vi "CPU_IRQ_handle.vi"(11 "registers":T1 {"P" format="%08b"; "PC" format="%04x"; "SP" format="%02x"; "Y" format="%02x"; "X" format="%02x"; "A" format="%02x"}) -> (3 "registers":T1 {"P" format="%08b"; "PC" format="%04x"; "SP" format="%02x"; "Y" format="%02x"; "X" format="%02x"; "A" format="%02x"})   [LabVIEW 2018]
uses:
  CPU_registers.ctl
  CIA/CIA_IRQ_oper.ctl
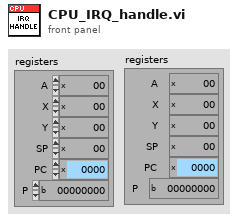
[diagram p1: front panel]
types:
  T1 = typedef "CPU_registers.ctl" = cluster{"A":u8, "X":u8, "Y":u8, "SP":u8, "PC":u16, "P":u8}
  T2 = typedef "CIA_IRQ_oper.ctl" = enum16{"init", "set mask", "set flag", "check active", "read reg"}
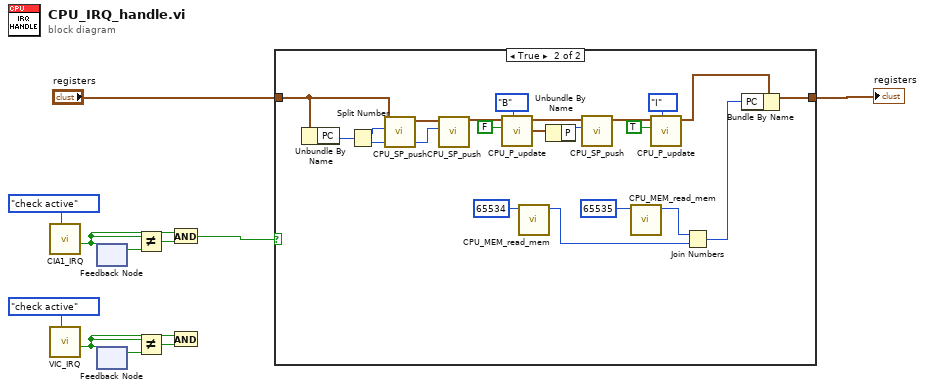
[diagram p0: block diagram]
diagram:
  n1 = call "CIA1_IRQ.vi"("oper"=CIA_IRQ_oper."check active") -> ("IRQ.active"=w2:bool)  [unwired: 8 in, 2 out]
  n2 = call "VIC_IRQ.vi"("oper"=CIA_IRQ_oper."check active") -> ("IRQ.active"=w6:bool)  [unwired: 8 in, 2 out]
  n3 = feedback-in #1(w2) -> ()
  n4 = feedback #1() -> (w10:bool)  [unwired: 1 in]
  n5 = feedback #2() -> (w4:bool)  [unwired: 1 in]
  n6 = feedback-in #2(w6) -> ()
  n7 = Not Equal?(x=w2, y=w10) -> (x != y?=w9:bool)
  n8 = Not Equal?(x=w6, y=w4) -> (x != y?=w5:bool)
  n9 = And(x=w2, y=w9) -> (x .and. y?=w1:bool)
  n10 = And(x=w6, y=w5) -> ()  [unwired: 1 out]
  n11 = case shown="True" w1 {
    tunnel: "registers" -> [w12 w27]
    tunnel: [w12 w14] -> w7
    frame False {
    }
    frame True {
      n12 = Unbundle By Name(w27) -> ("PC"=w32:u16)
      n13 = Split Number(x=w32) -> (hi(x)=w31:u8, lo(x)=w29:u8)
      n14 = call "CPU_SP_push.vi"("value"=w31, "registers"=w27) -> ("registers"=w30:T1)  [unwired: 9 in]
      n15 = call "CPU_SP_push.vi"("value"=w29, "registers"=w30) -> ("registers"=w24:T1)  [unwired: 9 in]
      n16 = call "CPU_P_update.vi"("flag"=enum8{"C", "Z", "I", "D", "B", "V", "N"}."B", "Value"=FALSE, "registers"=w24) -> ("registers"=w23:T1)  [unwired: 8 in]
      n17 = call "CPU_MEM_read_mem.vi"("address"=u16 65534) -> ("value out"=w19:u8)  [unwired: 10 in]
      n18 = Unbundle By Name(w23) -> ("P"=w25:u8)
      n19 = call "CPU_SP_push.vi"("value"=w25, "registers"=w23) -> ("registers"=w20:T1)  [unwired: 9 in]
      n20 = call "CPU_MEM_read_mem.vi"("address"=u16 65535) -> ("value out"=w18:u8)  [unwired: 10 in]
      n21 = call "CPU_P_update.vi"("flag"=enum8{"C", "Z", "I", "D", "B", "V", "N"}."I", "Value"=TRUE, "registers"=w20) -> ("registers"=w15:T1)  [unwired: 8 in]
      n22 = Join Numbers(hi=w18, lo=w19) -> ((hi.lo)=w13:u16)
      n23 = Bundle By Name(cluster=w15, "PC"=w13) -> (w14:T1)
    }
  }
  "registers" <- w7
